vi "Util_Waypoint_To_CubicInput.vi"(11 "WayPoints":T4[](array[typedef]) {"ANGLE" format="%13.3f"; "Y" format="%13.3f"; "X" format="%13.3f"}) -> (1 "Final POSE":T2 {"ROTATION"."SIN" format="%13.4f"; "ROTATION"."COS" format="%13.4f"; "ROTATION"."VALUE" format="%13.4f"; "TRANSLATION"."Y" format="%14.3f"; "TRANSLATION"."X" format="%14.3f"}, 2 "Internal Cubic Waypoints":T1[](array[typedef]) {"Y" format="%14.3f"; "X" format="%14.3f"}, 3 "Initial POSE":T2 {"ROTATION"."SIN" format="%13.4f"; "ROTATION"."COS" format="%13.4f"; "ROTATION"."VALUE" format="%13.4f"; "TRANSLATION"."Y" format="%14.3f"; "TRANSLATION"."X" format="%14.3f"})   [LabVIEW 2019, in "Trajectory_Library.lvlib"]
doc: "Utility function to convert utility waypoints to the input data structures needed to calculate cubic splines."
uses:
  Trajectory_Library.lvlib
  UTIL_WAYPOINT.ctl
  POSE2D.ctl
  TRANSLATION2D.ctl
  ROTATION2D.ctl
  Rotation_CreateAngle.vi
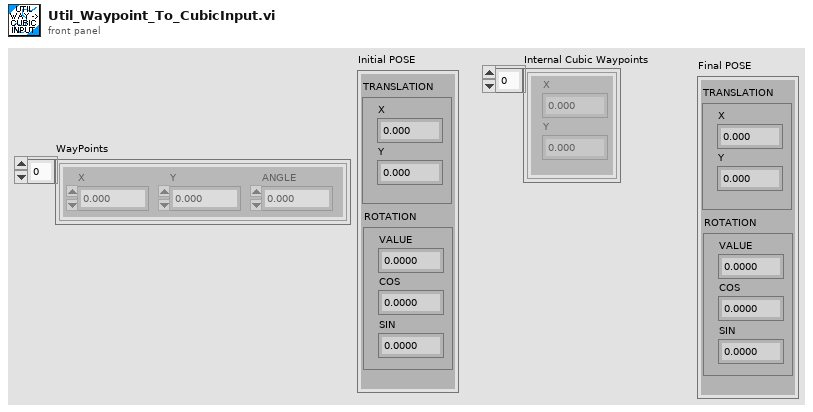
[diagram p1: front panel]
types:
  T1 = typedef "Trajectory_Library.lvlib/TRANSLATION2D.ctl" = cluster{"X":dbl, "Y":dbl}
  T2 = typedef "Trajectory_Library.lvlib/POSE2D.ctl" = cluster{"TRANSLATION":T1, "ROTATION":T3}
  T3 = typedef "Trajectory_Library.lvlib/ROTATION2D.ctl" = cluster{"VALUE":dbl, "COS":dbl, "SIN":dbl}
  T4 = typedef "Trajectory_Library.lvlib/UTIL_WAYPOINT.ctl" = cluster{"X":dbl, "Y":dbl, "ANGLE":dbl}
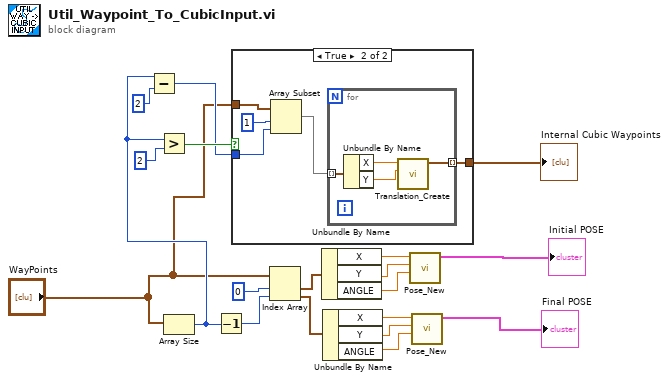
[diagram p0: block diagram]
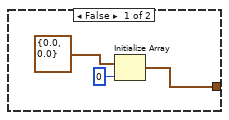
[diagram p2: hidden frame]
diagram:
  n1 = Array Size(array="WayPoints") -> (size(s)=w7:i32)
  n2 = Subtract(x=w7, y=2) -> (x-y=w5:i32)
  n3 = Greater?(x=w7, y=2) -> (0:w8:bool)
  n4 = Decrement(x=w7) -> (x-1=w18:i32)
  n5 = case shown="True" w8 {
    tunnel: [w20 w27] -> w1
    tunnel: "WayPoints" -> [_ w26]
    tunnel: w5 -> [_ w24]
    frame False {
      n6 = Initialize Array(T1 {"X"=0.0, "Y"=0.0} ("TRANSLATION"), 0 ("dimension size")) -> (w20:T1[])
    }
    frame True {
      n7 = Array Subset(array=w26, index=1, length=w24) -> (w23:T4[])
      n8 = for {
        tunnel: [w31] -> w27 mode=indexing
        tunnel: w23 -> [w30] mode=indexing
        n9 = Unbundle By Name(w30) -> ("X"=w29:dbl, "Y"=w28:dbl)
        n10 = call "Translation_Create.vi"("Y"=w28, "X"=w29) -> ("TRANSLATION"=w31:T1)  [unwired: 9 in]
      }
    }
  }
  "Internal Cubic Waypoints" <- w1
  n11 = Index Array(array="WayPoints", index #1=0 ("index"), index #2=w18) -> (element #1=w17:T4, element #2=w16:T4)
  n12 = Unbundle By Name(w17) -> ("X"=w15:dbl, "Y"=w14:dbl, "ANGLE"=w13:dbl)
  n13 = Unbundle By Name(w16) -> ("X"=w12:dbl, "Y"=w11:dbl, "ANGLE"=w10:dbl)
  n14 = call "Pose_New.vi"("Heading"=w13, "Y"=w14, "X"=w15) -> ("out POSe"=→"Initial POSE":T2)  [unwired: 8 in]
  n15 = call "Pose_New.vi"("Heading"=w10, "Y"=w11, "X"=w12) -> ("out POSe"=→"Final POSE":T2)  [unwired: 8 in]
